vi "Analyze (static).vi"(8 "error in (no error)":errorcluster, 9 "Energy":dbl[unit], 10 "Image in":T1, 11 "Analyze Fluence in":refnum<class "Analyze Fluence.lvclass">) -> (0 "error out":errorcluster, 1 "Result":refnum<class "Analyze Results Fluence.lvclass">, 2 "Image out":T1, 3 "Analyze Fluence out":refnum<class "Analyze Fluence.lvclass">)   [LabVIEW 2014, in "Analyze.lvlib" / "Analyze Fluence.lvclass"]
uses:
  Analyze Fluence.lvclass
  <vilib>/vision/Image Controls.llb/IMAQ Image.ctl
  Results and Overlays/Results Fluence/Analyze Results Fluence.lvclass
  Analyze Parameter/Analyze Parameter Energy/Analyze Parameter Energy.lvclass
  Analyze Parameter/Analyze Parameter Energy/Analyze Parameter Energy.lvclass/Analyze Parameter Energy.ctl
  Analyze Parameter/Analyze Parameter Energy/Write Energy.vi
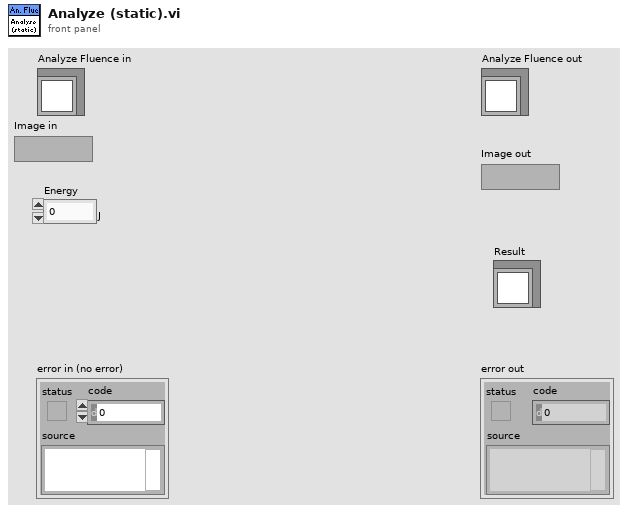
[diagram p1: front panel]
types:
  T1 = typedef "IMAQ Image.ctl" = refnum<image>
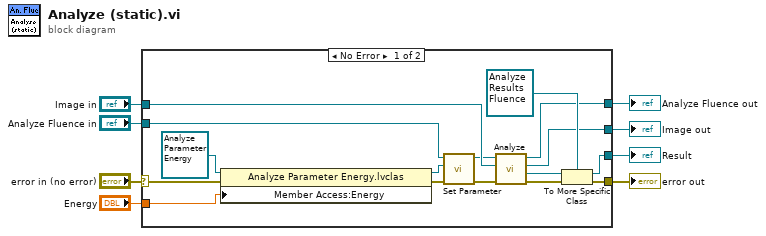
[diagram p0: block diagram]
diagram:
  n1 = case shown="No Error" "error in (no error)" {
    selector: "error in (no error)" -> [w9 w25]
    tunnel: "Analyze Fluence in" -> [w23 w27]
    tunnel: [w22 w27] -> w7
    tunnel: "Image in" -> [w21 w26]
    tunnel: [w18 _] -> w5
    tunnel: "Energy" -> [w16 _]
    tunnel: [w10 w25] -> w3
    tunnel: [w19 w26] -> w1
    frame No Error {
      n2 = property class="Analyze Parameter Energy.lvclas"(reference=refnum<class "Analyze Parameter Energy.lvclass"> refnum ("Analyze Parameter Energy.lvclass"), error in=w9, "Member Access:Energy"=w16) -> (reference out=w14:refnum<class "Analyze Parameter Energy.lvclass">, error out=w13:errorcluster)
      n3 = call-dynamic "Set Parameter.vi"("error in (no error)"=w13, "Analyze Parameter"=w14, "Analyze BaseClass in"=w23) -> ("error out"=w12:errorcluster, "Analyze BaseClass out"=w15:refnum<class "Analyze Fluence.lvclass">)  [unwired: 7 in]
      n4 = call-dynamic "Analyze.vi"("error in (no error)"=w12, "Image in"=w21, "Analyze Fluence in"=w15) -> ("error out"=w11:errorcluster, "Result"=w20:refnum<class "Analyze Results Base.lvclass">, "Image out"=w19:T1, "Analyze Fluence out"=w22:refnum<class "Analyze Fluence.lvclass">)  [unwired: 5 in]
      n5 = To More Specific Class(target class=refnum<class "Analyze Results Fluence.lvclass"> refnum ("Analyze Results Fluence.lvclass"), reference=w20, error in=w11) -> (specific class reference=w18:refnum<class "Analyze Results Fluence.lvclass">, error out=w10:errorcluster)
    }
    frame Error {
    }
  }
  "error out" <- w3
  "Analyze Fluence out" <- w7
  "Result" <- w5
  "Image out" <- w1
